vi "InitVNA (SubVI).vi"(0 "Start Freq. (MHz)":string="3000", 1 "Stop Freq. (MHz)":string, 5 "IFBW":string, 7 "Output Power":string, 9 "bus":i32, 11 "Number of Points":string, 12 "address":i16) -> (2 "Forced  Output Power":string, 3 "Instrument ID":string, 4 "Forced Sweep Time":string, 6 "Forced Number of Points":string, 8 "Forced IFBW":string, 10 "Freq. Array":dbl[](array[numeric]), 13 "Forced Start Freq.":string, 14 "Forced Stop Freq.":string, 15 "error out":errorcluster)   [LabVIEW 2013]
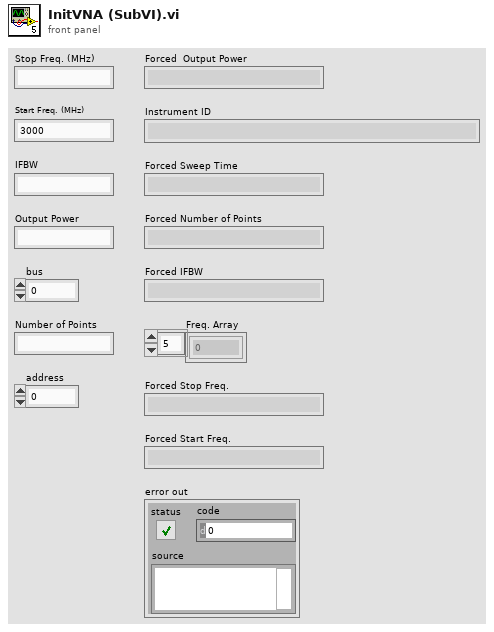
[diagram p1: front panel]
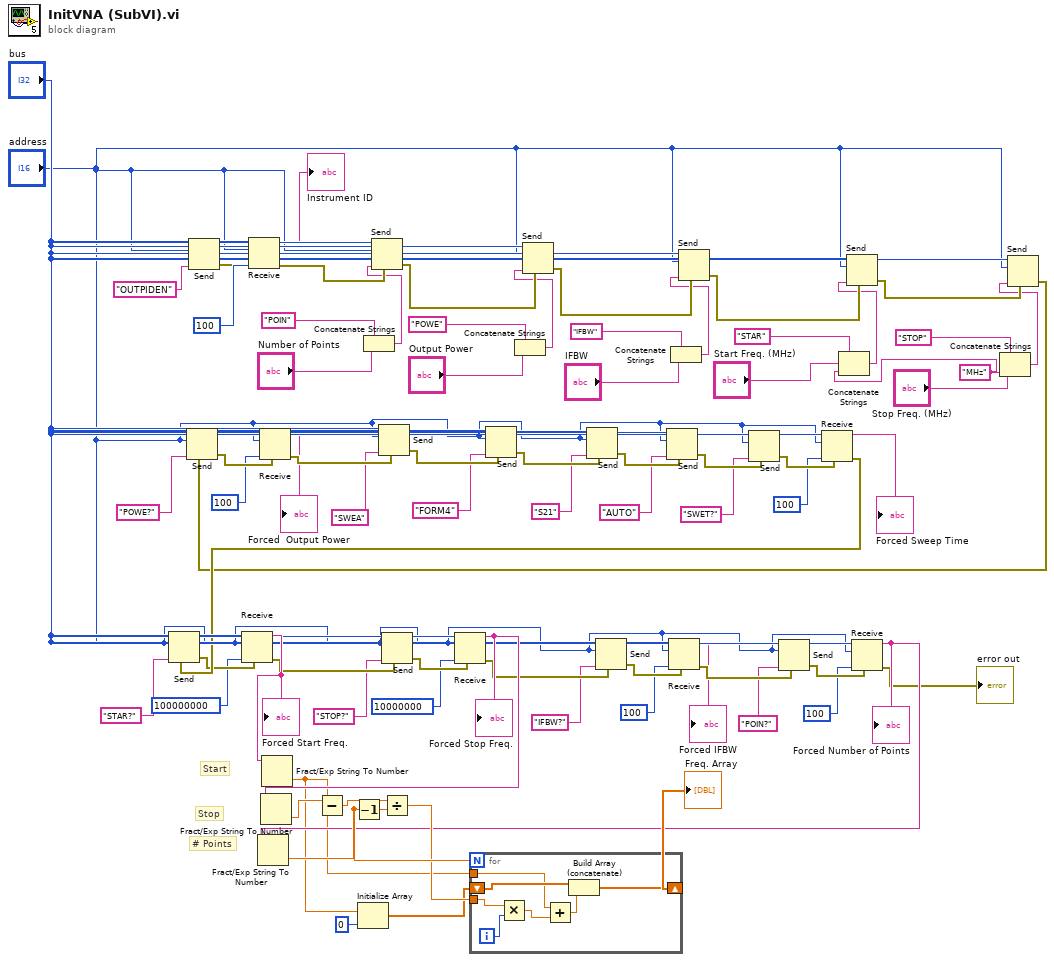
[diagram p0: block diagram]
diagram:
  w63 = "MHz" ("string")
  # "# Points"
  # "Stop"
  # "Start"
  n1 = Send(0:"bus", 2:"address", 5:"OUTPIDEN" ("data string")) -> (8:w5:errorcluster)  [unwired: 2 in, 2 out]
  n2 = Receive(4:w5, 6:100 ("count"), 8:"address", 9:"bus") -> (0:w10:errorcluster, 3:→"Instrument ID":string)  [unwired: 1 in, 2 out]
  n3 = Concatenate Strings("POIN" ("string"), "Number of Points") -> (w9:string)
  n4 = Send(0:"bus", 2:"address", 4:w10, 5:w9) -> (8:w22:errorcluster)  [unwired: 1 in, 2 out]
  n5 = Concatenate Strings("POWE" ("string"), "Output Power") -> (w13:string)
  n6 = Send(0:"bus", 2:"address", 4:w22, 5:w13) -> (8:w23:errorcluster)  [unwired: 1 in, 2 out]
  n7 = Concatenate Strings("IFBW" ("string"), "IFBW") -> (w16:string)
  n8 = Send(0:"bus", 2:"address", 4:w23, 5:w16) -> (8:w24:errorcluster)  [unwired: 1 in, 2 out]
  n9 = Concatenate Strings("STAR" ("string"), "Start Freq. (MHz)", w63) -> (w18:string)
  n10 = Send(0:"bus", 2:"address", 4:w24, 5:w18) -> (8:w25:errorcluster)  [unwired: 1 in, 2 out]
  n11 = Concatenate Strings("STOP" ("string"), "Stop Freq. (MHz)", w63) -> (w21:string)
  n12 = Send(0:"bus", 2:"address", 4:w25, 5:w21) -> (8:w57:errorcluster)  [unwired: 1 in, 2 out]
  n13 = Send(0:"bus", 2:"address", 4:w57, 5:"POWE?" ("data string")) -> (8:w56:errorcluster)  [unwired: 1 in, 2 out]
  n14 = Receive(4:w56, 6:100 ("count"), 8:"address", 9:"bus") -> (0:w58:errorcluster, 3:→"Forced  Output Power":string)  [unwired: 1 in, 2 out]
  n15 = Send(0:"bus", 2:"address", 4:w58, 5:"SWEA" ("string")) -> (8:w34:errorcluster)  [unwired: 1 in, 2 out]
  n16 = Send(0:"bus", 2:"address", 4:w34, 5:"FORM4" ("data string")) -> (8:w35:errorcluster)  [unwired: 1 in, 2 out]
  n17 = Send(0:"bus", 2:"address", 4:w35, 5:"S21" ("data string")) -> (8:w36:errorcluster)  [unwired: 1 in, 2 out]
  n18 = Send(0:"bus", 2:"address", 4:w36, 5:"AUTO" ("data string")) -> (8:w37:errorcluster)  [unwired: 1 in, 2 out]
  n19 = Send(0:"bus", 2:"address", 4:w37, 5:"SWET?" ("data string")) -> (8:w38:errorcluster)  [unwired: 1 in, 2 out]
  n20 = Receive(4:w38, 6:100 ("count"), 8:"address", 9:"bus") -> (0:w59:errorcluster, 3:→"Forced Sweep Time":string)  [unwired: 1 in, 2 out]
  n21 = Send(0:"bus", 2:"address", 4:w59, 5:"STAR?" ("data string")) -> (8:w41:errorcluster)  [unwired: 1 in, 2 out]
  n22 = Receive(4:w41, 6:100000000 ("count"), 8:"address", 9:"bus") -> (0:w60:errorcluster, 3:w67:string)  [unwired: 1 in, 2 out]
  "Forced Start Freq." <- w67
  n23 = Fract/Exp String To Number(string=w67) -> (number=w2:dbl)  [unwired: 3 in, 1 out]
  n24 = Initialize Array(w2, 0 ("dimension size")) -> (w1:dbl[])
  n25 = Send(0:"bus", 2:"address", 4:w60, 5:"STOP?" ("data string")) -> (8:w44:errorcluster)  [unwired: 1 in, 2 out]
  n26 = Receive(4:w44, 6:10000000 ("count"), 8:"address", 9:"bus") -> (0:w61:errorcluster, 3:w68:string)  [unwired: 1 in, 2 out]
  "Forced Stop Freq." <- w68
  n27 = Fract/Exp String To Number(string=w68) -> (number=w70:dbl)  [unwired: 3 in, 1 out]
  n28 = Subtract(x=w70, y=w2) -> (x-y=w71:dbl)
  n29 = Send(0:"bus", 2:"address", 4:w61, 5:"IFBW?" ("data string")) -> (8:w48:errorcluster)  [unwired: 1 in, 2 out]
  n30 = Receive(4:w48, 6:100 ("count"), 8:"address", 9:"bus") -> (0:w52:errorcluster, 3:→"Forced IFBW":string)  [unwired: 1 in, 2 out]
  n31 = Send(0:"bus", 2:"address", 4:w52, 5:"POIN?" ("data string")) -> (8:w51:errorcluster)  [unwired: 1 in, 2 out]
  n32 = Receive(4:w51, 6:100 ("count"), 8:"address", 9:"bus") -> (0:→"error out":errorcluster, 3:w69:string)  [unwired: 1 in, 2 out]
  "Forced Number of Points" <- w69
  n33 = Fract/Exp String To Number(string=w69) -> (number=w74:dbl)  [unwired: 3 in, 1 out]
  n34 = Decrement(x=w74) -> (x-1=w73:dbl)
  n35 = Divide(x=w71, y=w73) -> (x/y=w72:dbl)
  n36 = for {
    N: w74 -> [_]
    shift-right: [w81] -> w75
    shift-left: w1 -> [w82]
    tunnel: w72 -> [w78]
    tunnel: w2 -> [w79]
    i -> [w77]
    n37 = Multiply(x=w78, y=w77) -> (x*y=w76:dbl)
    n38 = Add(x=w79, y=w76) -> (x+y=w80:dbl)
    n39 = Build Array (concatenate)(w82, w80) -> (w81:dbl[])
  }
  "Freq. Array" <- w75
